vi "StreamHoldOn.vi"(8 "error in (no error)":errorcluster, 10 "StreamHoldOn":bool, 11 "IMAQdx Actor in":refnum<class "IMAQdx Actor.lvclass">) -> (0 "error out":errorcluster, 3 "IMAQdx Actor out":refnum<class "IMAQdx Actor.lvclass">)   [LabVIEW 2020]
uses:
  IMAQdx Actor.lvclass
  C:/Users/AlexK/work/LabVIEW Programme/POLARIS CAM Log Abw und E/Submodules/HIJ Vision/Camera Actors/Camera Actor/Camera Actor/Camera Actor.lvclass
  Camera Actor/Camera Actor/Camera Actor.lvclass/Camera Actor.ctl
  IMAQdx Actor.lvclass/IMAQdx Actor.ctl
  <resource>/objmgr/imaqdx.rc
  Camera Actor/Camera Actor/Camera Actor.lvclass
  C:/Program Files (x86)/National Instruments/LabVIEW 2020/vi.lib/ActorFramework/Actor/Actor.lvclass
  C:/Users/AlexK/work/LabVIEW Programme/POLARIS CAM Log Abw und E/Submodules/HIJ Vision/Camera Actors/IMAQdx Actor/IMAQdx Actor/IMAQdx Actor.lvclass
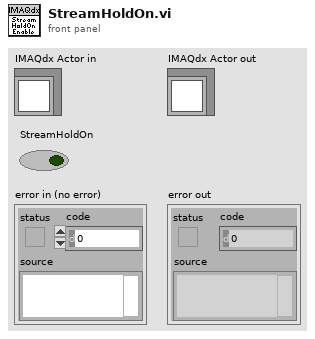
[diagram p1: front panel]
types:
  T1 = typedef "Camera Actor.lvlib/Camera Actor.lvclass/Operation Mode.ctl" = enum16{"Run", "Stop", "Exit", "Error", "Restart"}
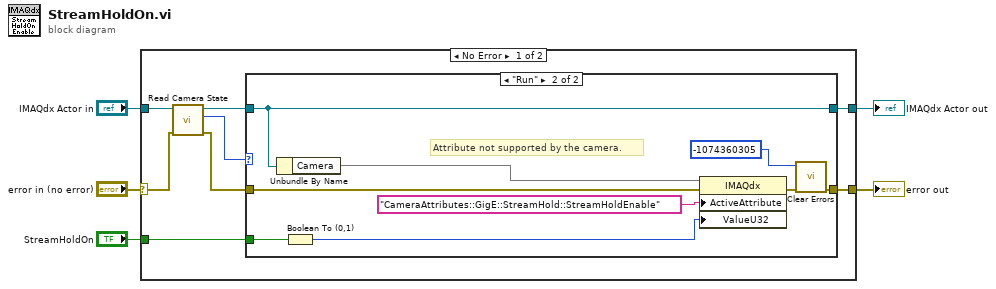
[diagram p0: block diagram]
diagram:
  n1 = case shown="No Error" "error in (no error)" {
    selector: "error in (no error)" -> [w9 w26]
    tunnel: "StreamHoldOn" -> [w13 _]
    tunnel: [w11 w26] -> w3
    tunnel: "IMAQdx Actor in" -> [w12 w25]
    tunnel: [w6 w25] -> w1
    frame No Error {
      n2 = call "Read Camera State.vi"("error in (no error)"=w9, "Camera Actor in"=w12) -> ("error out"=w8:errorcluster, "Operation Mode"=w7:T1, "Camera Actor out"=w10:refnum<class "IMAQdx Actor.lvclass">)  [unwired: 7 in]
      n3 = case shown="\"Run\"" w7 {
        tunnel: w13 -> [_ w21]
        tunnel: [w14 w19] -> w11
        tunnel: w10 -> [w15 w16]
        tunnel: w8 -> [w14 w17]
        tunnel: [w15 w16] -> w6
        frame "Error", Default {
        }
        frame "Run" {
          # "Attribute not supported by the camera."
          n4 = Unbundle By Name(w16) -> ("Camera"=w23)
          n5 = Boolean To (0,1)(Boolean=w21) -> (0, 1=w24:i16)
          n6 = property class="IMAQdx"(reference=w23, error in=w17, "ActiveAttribute"="CameraAttributes::GigE::StreamHold::StreamHoldEnable", "ValueU32"=w24) -> (error out=w20:errorcluster)  [unwired: 1 out]
          n7 = call <vilib>:"Clear Errors.vi"("error in (no error)"=w20, "specific error code to clear (0: all)"=-1074360305) -> ("error out"=w19:errorcluster)  [unwired: 4 in, 1 out]
        }
      }
    }
    frame Error {
    }
  }
  "error out" <- w3
  "IMAQdx Actor out" <- w1
